vi "Run Panel.vi"(8 "error in (no error)":errorcluster, 10 "Panel":refnum<class "Panel.lvclass">, 11 "PanelManager in":refnum<class "PanelManager.lvclass">) -> (0 "error out":errorcluster, 3 "PanelManager out":refnum<class "PanelManager.lvclass">)   [LabVIEW 2018, in "OOPanel.lvlib" / "PanelManager.lvclass"]
uses:
  PanelManager.lvclass
  Panel/Panel.lvclass
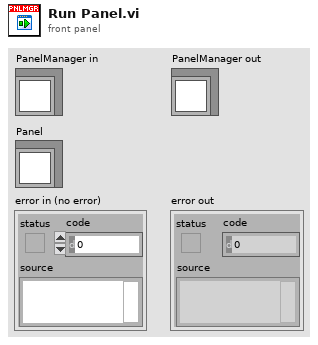
[diagram p1: front panel]
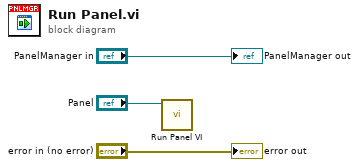
[diagram p0: block diagram]
diagram:
  n1 = call "Run Panel VI.vi"("Panel in"="Panel") -> ()  [unwired: 9 in, 2 out]
  "error out" <- "error in (no error)"
  "PanelManager out" <- "PanelManager in"
